vi "Parse Time.vi"(8 "error in (no error)":errorcluster, 11 "data":string) -> (0 "error out":errorcluster, 3 "Time Stamp":timestamp)   [LabVIEW 2018]
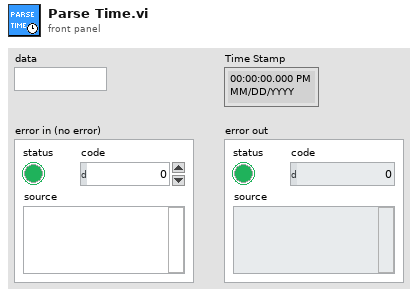
[diagram p1: front panel]
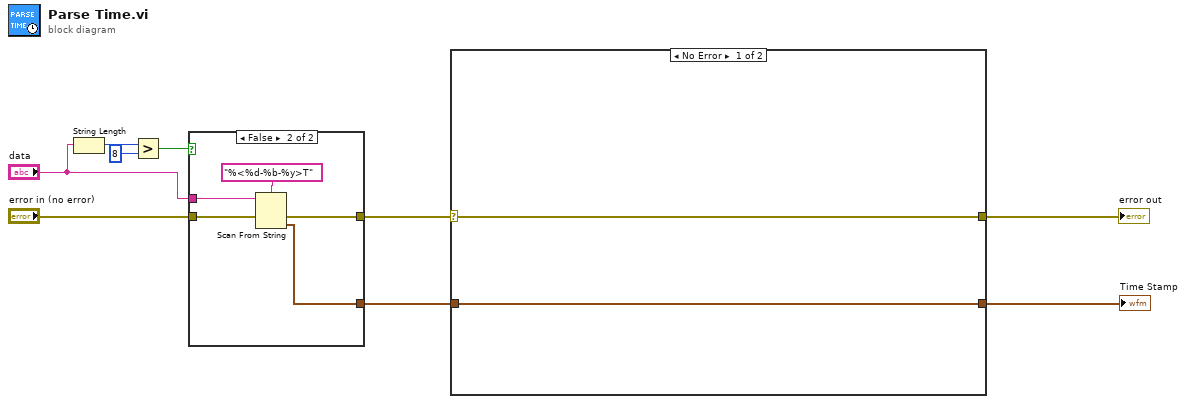
[diagram p0: block diagram]
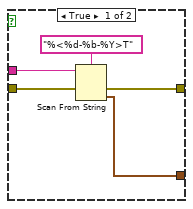
[diagram p2: hidden frame]
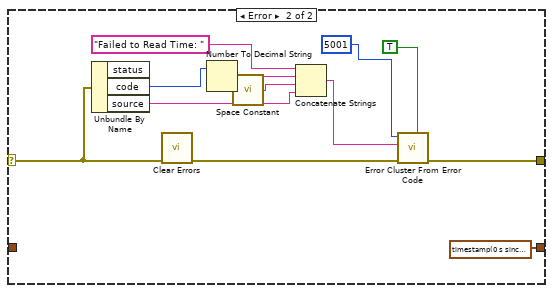
[diagram p3: hidden frame]
diagram:
  n1 = String Length(string="data") -> (length=w4:i32)
  n2 = Greater?(x=w4, y=8) -> (0:w1:bool)
  n3 = case shown="False" w1 {
    tunnel: "error in (no error)" -> [w14 w19]
    tunnel: [w12 w17] -> w8
    tunnel: [w11 w16] -> w5
    tunnel: "data" -> [w10 w15]
    frame True {
      n4 = Scan From String(format string="%<%d-%b-%Y>T", input string=w10, error in=w14) -> (error out=w12:errorcluster, output 1=w11:timestamp)  [unwired: 2 in, 2 out]
    }
    frame False {
      n5 = Scan From String(format string="%<%d-%b-%y>T", input string=w15, error in=w19) -> (error out=w17:errorcluster, output 1=w16:timestamp)  [unwired: 2 in, 2 out]
    }
  }
  n6 = case shown="No Error" w8 {
    selector: w8 -> [w21 w29]
    tunnel: [w21 w31] -> w7
    tunnel: [w20 timestamp(0 s since 1904-01-01)] -> w6
    tunnel: w5 -> [w20 _]
    frame No Error {
    }
    frame Error {
      n7 = Unbundle By Name(w29) -> ("code"=w26:i32, "source"=w25:string)  [unwired: 1 out]
      n8 = call <vilib>:"Clear Errors.vi"("error in (no error)"=w29) -> ("error out"=w30:errorcluster)  [unwired: 5 in, 1 out]
      n9 = Number To Decimal String(number=w26) -> (decimal integer string=w23:string)  [unwired: 1 in]
      n10 = call <vilib>:"Space Constant.vi"() -> ("String"=w24:string)
      n11 = Concatenate Strings("Failed to Read Time: " ("error message (\"\")"), w23, w24, w25) -> (w22:string)
      n12 = call <vilib>:"Error Cluster From Error Code.vi"("is warning? (False)"=TRUE, "error in (no error)"=w30, "error message (\"\")"=w22, "error code (0)"=5001) -> ("error out"=w31:errorcluster)  [unwired: 5 in]
    }
  }
  "error out" <- w7
  "Time Stamp" <- w6
